vi "Dependencies.vi"   [LabVIEW 2009]
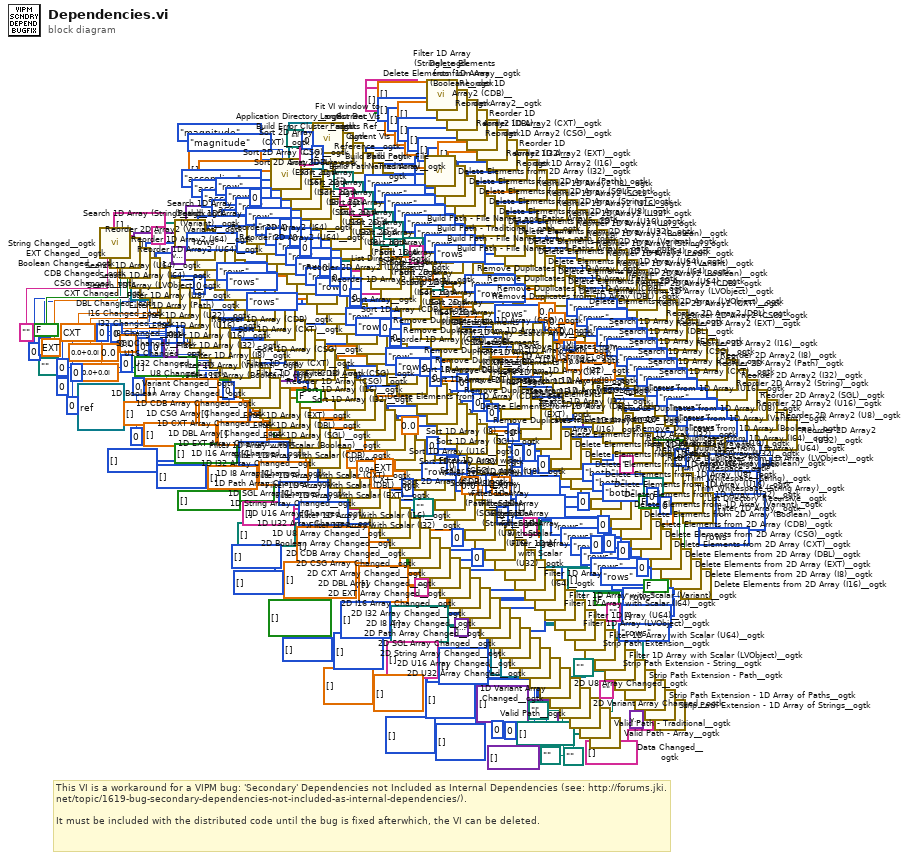
[diagram p0: block diagram]
diagram:
  # "This VI is a workaround for a VIPM bug: 'Secondary' Dependencies not Included as Internal Dependencies (see: http://forums.jki.net/topic/1619-bug-secondary-dependencies-not-included-as-internal-dependencies/).\n\nIt must be included with the distributed code until the bug is fixed afterwhich, the VI can be deleted."
  n1 = call <userlib>:"String Changed__ogtk.vi"("String"="") -> ()  [unwired: 1 out]
  n2 = call <userlib>:"EXT Changed__ogtk.vi"("EXT"=ext 0.0) -> ()  [unwired: 1 out]
  n3 = call <userlib>:"Boolean Changed__ogtk.vi"("Boolean"=FALSE) -> ()  [unwired: 1 out]
  n4 = call <userlib>:"CDB Changed__ogtk.vi"("CDB"=cdb 0.0+0.0i) -> ()  [unwired: 1 out]
  n5 = call <userlib>:"CSG Changed__ogtk.vi"("CSG"=csg 0.0+0.0i) -> ()  [unwired: 1 out]
  n6 = call <userlib>:"CXT Changed__ogtk.vi"("CXT"=cxt 0.0+0.0i) -> ()  [unwired: 1 out]
  n7 = call <userlib>:"DBL Changed__ogtk.vi"("DBL"=0.0) -> ()  [unwired: 1 out]
  n8 = call <userlib>:"I16 Changed__ogtk.vi"("I16"=i16 0) -> ()  [unwired: 1 out]
  n9 = call <userlib>:"Search 1D Array (String)__ogtk.vi"("Array"=string[] [], "Element Data"="", "Start Index (0)"=0) -> ()  [unwired: 6 in, 1 out]
  n10 = call <userlib>:"I32 Changed__ogtk.vi"("I32"=0) -> ()  [unwired: 1 out]
  n11 = call <userlib>:"Search 1D Array (Path)__ogtk.vi"("Array"=path[] [], "Element Data"=path "", "Start Index (0)"=0) -> ()  [unwired: 6 in, 1 out]
  n12 = call <userlib>:"I8 Changed__ogtk.vi"("I8"=i8 0) -> ()  [unwired: 1 out]
  n13 = call <userlib>:"Search 1D Array (Variant)__ogtk.vi"("Array"=variant[] [], "Element Data"=variant, "Start Index (0)"=0) -> ()  [unwired: 6 in, 1 out]
  n14 = call <userlib>:"SGL Changed__ogtk.vi"("SGL"=sgl 0.0) -> ()  [unwired: 1 out]
  n15 = call <userlib>:"Search 1D Array (U64)__ogtk.vi"("Array"=u64[] [], "Element Data"=u64 0, "Start Index (0)"=0) -> ()  [unwired: 6 in, 1 out]
  n16 = call <userlib>:"U16 Changed__ogtk.vi"("U16"=u16 0) -> ()  [unwired: 1 out]
  n17 = call <userlib>:"Search 1D Array (I64)__ogtk.vi"("Array"=i64[] [], "Element Data"=i64 0, "Start Index (0)"=0) -> ()  [unwired: 6 in, 1 out]
  n18 = call <userlib>:"U32 Changed__ogtk.vi"("U32"=u32 0) -> ()  [unwired: 1 out]
  n19 = call <userlib>:"Search 1D Array (LVObject)__ogtk.vi"("Array"=refnum<class>[] [], "Element Data"=refnum<class> refnum, "Start Index (0)"=0) -> ()  [unwired: 6 in, 1 out]
  n20 = call <userlib>:"U8 Changed__ogtk.vi"("U8"=u8 0) -> ()  [unwired: 1 out]
  n21 = call <userlib>:"Filter 1D Array (U8)__ogtk.vi"("items to filter"=u8[] [], "array"=u8[] []) -> ()  [unwired: 4 in, 2 out]
  n22 = call <userlib>:"Variant Changed__ogtk.vi"("Variant"=variant) -> ()  [unwired: 1 out]
  n23 = call <userlib>:"Filter 1D Array (Path)__ogtk.vi"("items to filter"=path[] [], "array"=path[] []) -> ()  [unwired: 4 in, 2 out]
  n24 = call <userlib>:"Reorder 2D Array2 (Variant)__ogtk.vi"("reorder (rows)"=enum16{"rows", "columns"}."rows", "indices"=i32[] [], "array"=variant[][] []) -> ()  [unwired: 8 in, 1 out]
  n25 = call <userlib>:"1D Boolean Array Changed__ogtk.vi"("1D Boolean Array"=bool[] []) -> ()  [unwired: 1 out]
  n26 = call <userlib>:"Filter 1D Array (U32)__ogtk.vi"("items to filter"=u32[] [], "array"=u32[] []) -> ()  [unwired: 4 in, 2 out]
  n27 = call <userlib>:"Reorder 1D Array2 (I64)__ogtk.vi"("indices"=i32[] [], "array"=i64[] []) -> ()  [unwired: 9 in, 1 out]
  n28 = call <userlib>:"1D CDB Array Changed__ogtk.vi"("1D CDB Array"=cdb[] []) -> ()  [unwired: 1 out]
  n29 = call <userlib>:"Filter 1D Array (U16)__ogtk.vi"("items to filter"=u16[] [], "array"=u16[] []) -> ()  [unwired: 4 in, 2 out]
  n30 = call <userlib>:"Reorder 1D Array2 (U64)__ogtk.vi"("indices"=i32[] [], "array"=u64[] []) -> ()  [unwired: 9 in, 1 out]
  n31 = call <userlib>:"1D CSG Array Changed__ogtk.vi"("1D CSG Array"=csg[] []) -> ()  [unwired: 1 out]
  n32 = call <userlib>:"Sort 2D Array (CXT)__ogtk.vi"("Column/Row to Sort By"=u32 0, "Method (magnitude)"=enum16{"real", "imaginary", "magnitude"}."magnitude", "Sort By in"=enum16{"row", "column"}."row", "Order"=enum16{"ascending", "descending"}."ascending", "Array in"=cxt[][] []) -> ()  [unwired: 3 in, 4 out]
  n33 = call <userlib>:"Filter 1D Array (I16)__ogtk.vi"("items to filter"=i16[] [], "array"=i16[] []) -> ()  [unwired: 4 in, 2 out]
  n34 = call <userlib>:"Reorder 2D Array2 (I64)__ogtk.vi"("reorder (rows)"=enum16{"rows", "columns"}."rows", "indices"=i32[] [], "array"=i64[][] []) -> ()  [unwired: 8 in, 1 out]
  n35 = call <userlib>:"1D CXT Array Changed__ogtk.vi"("1D CXT Array"=cxt[] []) -> ()  [unwired: 1 out]
  n36 = call <userlib>:"Sort 2D Array (CSG)__ogtk.vi"("Column/Row to Sort By"=u32 0, "Method (magnitude)"=enum16{"real", "imaginary", "magnitude"}."magnitude", "Sort By in"=enum16{"row", "column"}."row", "Order"=enum16{"ascending", "descending"}."ascending", "Array in"=csg[][] []) -> ()  [unwired: 3 in, 4 out]
  n37 = call <userlib>:"Filter 1D Array (I32)__ogtk.vi"("items to filter"=i32[] [], "array"=i32[] []) -> ()  [unwired: 4 in, 2 out]
  n38 = call <userlib>:"Reorder 2D Array2 (U64)__ogtk.vi"("reorder (rows)"=enum16{"rows", "columns"}."rows", "indices"=i32[] [], "array"=u64[][] []) -> ()  [unwired: 8 in, 1 out]
  n39 = call <userlib>:"1D DBL Array Changed__ogtk.vi"("1D DBL Array"=dbl[] []) -> ()  [unwired: 1 out]
  n40 = call <userlib>:"Sort 2D Array (DBL)__ogtk.vi"("Column/Row to Sort By"=u32 0, "Sort By in"=enum16{"row", "column"}."row", "Order"=enum16{"ascending", "descending"}."ascending", "Array in"=dbl[][] []) -> ()  [unwired: 4 in, 4 out]
  n41 = call <userlib>:"Filter 1D Array (I8)__ogtk.vi"("items to filter"=i8[] [], "array"=i8[] []) -> ()  [unwired: 4 in, 2 out]
  n42 = call <userlib>:"Reorder 1D Array2 (LVObject)__ogtk.vi"("indices"=i32[] [], "array"=refnum<class>[] []) -> ()  [unwired: 9 in, 1 out]
  n43 = call <userlib>:"1D EXT Array Changed__ogtk.vi"("1D EXT Array"=ext[] []) -> ()  [unwired: 1 out]
  n44 = call <userlib>:"Sort 2D Array (EXT)__ogtk.vi"("Column/Row to Sort By"=u32 0, "Sort By in"=enum16{"row", "column"}."row", "Order"=enum16{"ascending", "descending"}."ascending", "Array in"=ext[][] []) -> ()  [unwired: 4 in, 4 out]
  n45 = call <userlib>:"Filter 1D Array (Variant)__ogtk.vi"("items to filter"=variant[] [], "array"=variant[] []) -> ()  [unwired: 4 in, 2 out]
  n46 = call <userlib>:"Reorder 2D Array2 (LVObject)__ogtk.vi"("reorder (rows)"=enum16{"rows", "columns"}."rows", "indices"=i32[] [], "array"=refnum<class>[][] []) -> ()  [unwired: 8 in, 1 out]
  n47 = call <userlib>:"1D I16 Array Changed__ogtk.vi"("1D I16 Array"=i16[] []) -> ()  [unwired: 1 out]
  n48 = call <userlib>:"Sort 2D Array (I16)__ogtk.vi"("Column/Row to Sort By"=u32 0, "Sort By in"=enum16{"row", "column"}."row", "Order"=enum16{"ascending", "descending"}."ascending", "Array in"=i16[][] []) -> ()  [unwired: 4 in, 4 out]
  n49 = call <userlib>:"Application Directory__ogtk.vi"("Relative path (.)"=path "") -> ()  [unwired: 1 out]
  n50 = call <userlib>:"Filter 1D Array (Boolean)__ogtk.vi"("items to filter"=bool[] [], "array"=bool[] []) -> ()  [unwired: 4 in, 2 out]
  n51 = call-poly <userlib>:"Sort Array__ogtk.vi"("Order"=enum16{"ascending", "descending"}."ascending", "Array in"=dbl[] []) -> ()  [unwired: 8 in, 2 out]
  n52 = call <userlib>:"1D I32 Array Changed__ogtk.vi"("1D I32 Array"=i32[] []) -> ()  [unwired: 1 out]
  n53 = call <userlib>:"Sort 2D Array (I32)__ogtk.vi"("Column/Row to Sort By"=u32 0, "Sort By in"=enum16{"row", "column"}."row", "Order"=enum16{"ascending", "descending"}."ascending", "Array in"=i32[][] []) -> ()  [unwired: 4 in, 4 out]
  n54 = call <userlib>:"Build Error Cluster__ogtk.vi"("String to Prepend to source (\"\")"="" ("String to Prepend to source (\"\")"), "code"=0) -> ()  [unwired: 1 out]
  n55 = call <userlib>:"Filter 1D Array (CXT)__ogtk.vi"("items to filter"=cxt[] [], "array"=cxt[] []) -> ()  [unwired: 4 in, 2 out]
  n56 = call <userlib>:"Sort 1D Array (CDB)__ogtk.vi"("Method (magnitude)"=enum16{"real", "imaginary", "magnitude"}."magnitude", "Order"=enum16{"ascending", "descending"}."ascending", "Array in"=cdb[] []) -> ()  [unwired: 7 in, 2 out]
  n57 = call <userlib>:"1D I8 Array Changed__ogtk.vi"("1D I8 Array"=i8[] []) -> ()  [unwired: 1 out]
  n58 = call <userlib>:"Sort 2D Array (I8)__ogtk.vi"("Column/Row to Sort By"=u32 0, "Sort By in"=enum16{"row", "column"}."row", "Order"=enum16{"ascending", "descending"}."ascending", "Array in"=i8[][] []) -> ()  [unwired: 4 in, 4 out]
  n59 = call <userlib>:"Fit VI window to Largest Dec__ogtk.vi"("error in (no error)"=errorcluster {"status"=FALSE, "code"=0, "source"=""}, "border spacing (2 px)"=2, "VI Ref (calling VI)"=refnum<vi> refnum) -> ()  [unwired: 3 in, 2 out]
  n60 = call <userlib>:"Filter 1D Array (CDB)__ogtk.vi"("items to filter"=cdb[] [], "array"=cdb[] []) -> ()  [unwired: 4 in, 2 out]
  n61 = call <userlib>:"Reorder 1D Array (CDB)__ogtk.vi"("Sorted Pointers in"=i32[] [], "Array in"=cdb[] []) -> ()  [unwired: 8 in, 2 out]
  n62 = call <userlib>:"1D Path Array Changed__ogtk.vi"("1D Path Array"=path[] []) -> ()  [unwired: 1 out]
  n63 = call <userlib>:"Sort 2D Array (SGL)__ogtk.vi"("Column/Row to Sort By"=u32 0, "Sort By in"=enum16{"row", "column"}."row", "Order"=enum16{"ascending", "descending"}."ascending", "Array in"=sgl[][] []) -> ()  [unwired: 4 in, 4 out]
  n64 = call <userlib>:"Current VIs Parents Ref__ogtk.vi"() -> ()  [unwired: 2 in, 1 out]
  n65 = call <userlib>:"Filter 1D Array (CSG)__ogtk.vi"("items to filter"=csg[] [], "array"=csg[] []) -> ()  [unwired: 4 in, 2 out]
  n66 = call <userlib>:"Sort 1D Array (CXT)__ogtk.vi"("Method (magnitude)"=enum16{"real", "imaginary", "magnitude"}."magnitude", "Order"=enum16{"ascending", "descending"}."ascending", "Array in"=cxt[] []) -> ()  [unwired: 7 in, 2 out]
  n67 = call <userlib>:"1D SGL Array Changed__ogtk.vi"("1D SGL Array"=sgl[] []) -> ()  [unwired: 1 out]
  n68 = call <userlib>:"Sort 2D Array (U16)__ogtk.vi"("Column/Row to Sort By"=u32 0, "Sort By in"=enum16{"row", "column"}."row", "Order"=enum16{"ascending", "descending"}."ascending", "Array in"=u16[][] []) -> ()  [unwired: 4 in, 4 out]
  n69 = call <userlib>:"Current VIs Reference__ogtk.vi"() -> ()  [unwired: 5 in, 1 out]
  n70 = call <userlib>:"Filter 1D Array (EXT)__ogtk.vi"("items to filter"=ext[] [], "array"=ext[] []) -> ()  [unwired: 4 in, 2 out]
  n71 = call <userlib>:"Reorder 1D Array (CXT)__ogtk.vi"("Sorted Pointers in"=i32[] [], "Array in"=cxt[] []) -> ()  [unwired: 8 in, 2 out]
  n72 = call <userlib>:"1D String Array Changed__ogtk.vi"("1D String Array"=string[] []) -> ()  [unwired: 1 out]
  n73 = call <userlib>:"Sort 2D Array (U32)__ogtk.vi"("Column/Row to Sort By"=u32 0, "Sort By in"=enum16{"row", "column"}."row", "Order"=enum16{"ascending", "descending"}."ascending", "Array in"=u32[][] []) -> ()  [unwired: 4 in, 4 out]
  n74 = call-poly <userlib>:"Build Path__ogtk.vi"("name or relative path"="", "base path"=path "") -> ()  [unwired: 1 out]
  n75 = call <userlib>:"Filter 1D Array (DBL)__ogtk.vi"("items to filter"=dbl[] [], "array"=dbl[] []) -> ()  [unwired: 4 in, 2 out]
  n76 = call <userlib>:"Sort 1D Array (CSG)__ogtk.vi"("Method (magnitude)"=enum16{"real", "imaginary", "magnitude"}."magnitude", "Order"=enum16{"ascending", "descending"}."ascending", "Array in"=csg[] []) -> ()  [unwired: 7 in, 2 out]
  n77 = call <userlib>:"1D U16 Array Changed__ogtk.vi"("1D U16 Array"=u16[] []) -> ()  [unwired: 1 out]
  n78 = call <userlib>:"Sort 2D Array (U8)__ogtk.vi"("Column/Row to Sort By"=u32 0, "Sort By in"=enum16{"row", "column"}."row", "Order"=enum16{"ascending", "descending"}."ascending", "Array in"=u8[][] []) -> ()  [unwired: 4 in, 4 out]
  n79 = call <userlib>:"Build Path - Traditional__ogtk.vi"("name or relative path"="", "base path"=path "") -> ()  [unwired: 1 out]
  n80 = call <userlib>:"Filter 1D Array (SGL)__ogtk.vi"("items to filter"=sgl[] [], "array"=sgl[] []) -> ()  [unwired: 4 in, 2 out]
  n81 = call <userlib>:"Reorder 1D Array (CSG)__ogtk.vi"("Sorted Pointers in"=i32[] [], "Array in"=csg[] []) -> ()  [unwired: 8 in, 2 out]
  n82 = call <userlib>:"1D U32 Array Changed__ogtk.vi"("1D U32 Array"=u32[] []) -> ()  [unwired: 1 out]
  n83 = call <userlib>:"Sort 1D Array (Path)__ogtk.vi"("Order"=enum16{"ascending", "descending"}."ascending", "Array in"=path[] []) -> ()  [unwired: 8 in, 2 out]
  n84 = call <userlib>:"Build Path - File Names Array__ogtk.vi"("name or relative path"=string[] [], "base path"=path "") -> ()  [unwired: 1 out]
  n85 = call <userlib>:"Filter 1D Array with Scalar (Boolean)__ogtk.vi"("items to filter"=FALSE, "array"=bool[] []) -> ()  [unwired: 4 in, 2 out]
  n86 = call <userlib>:"Sort 1D Array (DBL)__ogtk.vi"("Order"=enum16{"ascending", "descending"}."ascending", "Array in"=dbl[] []) -> ()  [unwired: 8 in, 2 out]
  n87 = call <userlib>:"1D U8 Array Changed__ogtk.vi"("1D U8 Array"=u8[] []) -> ()  [unwired: 1 out]
  n88 = call <userlib>:"Sort 1D Array (String)__ogtk.vi"("Order"=enum16{"ascending", "descending"}."ascending", "Array in"=string[] []) -> ()  [unwired: 8 in, 2 out]
  n89 = call <userlib>:"Build Path - File Names and Paths Arrays__ogtk.vi"("name or relative path"=string[] [], "base path"=path[] []) -> ()  [unwired: 1 out]
  n90 = call <userlib>:"Filter 1D Array with Scalar (CDB)__ogtk.vi"("items to filter"=cdb 0.0+0.0i, "array"=cdb[] []) -> ()  [unwired: 4 in, 2 out]
  n91 = call <userlib>:"Sort 1D Array (EXT)__ogtk.vi"("Order"=enum16{"ascending", "descending"}."ascending", "Array in"=ext[] []) -> ()  [unwired: 8 in, 2 out]
  n92 = call <userlib>:"2D Boolean Array Changed__ogtk.vi"("2D Boolean Array"=bool[][] []) -> ()  [unwired: 1 out]
  n93 = call <userlib>:"Sort 2D Array (Path)__ogtk.vi"("Column/Row to Sort By"=u32 0, "Sort By in"=enum16{"row", "column"}."row", "Order"=enum16{"ascending", "descending"}."ascending", "Array in"=path[][] []) -> ()  [unwired: 4 in, 4 out]
  n94 = call <userlib>:"Build Path - Traditional - path__ogtk.vi"("name or relative path"=path "", "base path"=path "") -> ()  [unwired: 1 out]
  n95 = call <userlib>:"Filter 1D Array with Scalar (CSG)__ogtk.vi"("items to filter"=csg 0.0+0.0i, "array"=csg[] []) -> ()  [unwired: 4 in, 2 out]
  n96 = call <userlib>:"Sort 1D Array (I16)__ogtk.vi"("Order"=enum16{"ascending", "descending"}."ascending", "Array in"=i16[] []) -> ()  [unwired: 8 in, 2 out]
  n97 = call <userlib>:"2D CDB Array Changed__ogtk.vi"("2D CDB Array"=cdb[][] []) -> ()  [unwired: 1 out]
  n98 = call <userlib>:"Sort 2D Array (String)__ogtk.vi"("Column/Row to Sort By"=u32 0, "Sort By in"=enum16{"row", "column"}."row", "Order"=enum16{"ascending", "descending"}."ascending", "Array in"=string[][] []) -> ()  [unwired: 4 in, 4 out]
  n99 = call <userlib>:"Build Path - File Names Array - path__ogtk.vi"("name or relative path"=path[] [], "base path"=path "") -> ()  [unwired: 1 out]
  n100 = call <userlib>:"Filter 1D Array with Scalar (CXT)__ogtk.vi"("items to filter"=cxt 0.0+0.0i, "array"=cxt[] []) -> ()  [unwired: 4 in, 2 out]
  n101 = call <userlib>:"Sort 1D Array (I32)__ogtk.vi"("Order"=enum16{"ascending", "descending"}."ascending", "Array in"=i32[] []) -> ()  [unwired: 8 in, 2 out]
  n102 = call <userlib>:"2D CSG Array Changed__ogtk.vi"("2D CSG Array"=csg[][] []) -> ()  [unwired: 1 out]
  n103 = call <userlib>:"Sort 1D Array (I64)__ogtk.vi"("Order"=enum16{"ascending", "descending"}."ascending", "Array in"=i64[] []) -> ()  [unwired: 8 in, 2 out]
  n104 = call <userlib>:"Build Path - File Names and Paths Arrays - path__ogtk.vi"("name or relative path"=path[] [], "base path"=path[] []) -> ()  [unwired: 1 out]
  n105 = call <userlib>:"Delete Elements from 2D Array (I32)__ogtk.vi"("delete (rows or columns)"=enum16{"rows", "columns"}."rows", "indices"=i32[] [], "array"=i32[][] []) -> ()  [unwired: 7 in, 2 out]
  n106 = call <userlib>:"Filter 1D Array with Scalar (DBL)__ogtk.vi"("items to filter"=0.0, "array"=dbl[] []) -> ()  [unwired: 4 in, 2 out]
  n107 = call <userlib>:"Filter 1D Array (String)__ogtk.vi"("items to filter"=string[] [], "array"=string[] []) -> ()  [unwired: 4 in, 2 out]
  n108 = call <userlib>:"Sort 1D Array (I8)__ogtk.vi"("Order"=enum16{"ascending", "descending"}."ascending", "Array in"=i8[] []) -> ()  [unwired: 8 in, 2 out]
  n109 = call <userlib>:"2D CXT Array Changed__ogtk.vi"("2D CXT Array"=cxt[][] []) -> ()  [unwired: 1 out]
  n110 = call <userlib>:"Sort 1D Array (U64)__ogtk.vi"("Order"=enum16{"ascending", "descending"}."ascending", "Array in"=u64[] []) -> ()  [unwired: 8 in, 2 out]
  n111 = call <userlib>:"List Directory__ogtk.vi"("error in (no error)"=errorcluster {"status"=FALSE, "code"=0, "source"=""}, "pattern"="", "directory path"=path "") -> ()  [unwired: 1 in, 4 out]
  n112 = call <userlib>:"Delete Elements from 2D Array (Path)__ogtk.vi"("delete (rows or columns)"=enum16{"rows", "columns"}."rows", "indices"=i32[] [], "array"=path[][] []) -> ()  [unwired: 7 in, 2 out]
  n113 = call <userlib>:"Filter 1D Array with Scalar (EXT)__ogtk.vi"("items to filter"=ext 0.0, "array"=ext[] []) -> ()  [unwired: 4 in, 2 out]
  n114 = call-poly <userlib>:"Delete Elements from Array__ogtk.vi"("indices"=i32[] [], "array"=dbl[] []) -> ()  [unwired: 8 in, 2 out]
  n115 = call <userlib>:"Sort 1D Array (SGL)__ogtk.vi"("Order"=enum16{"ascending", "descending"}."ascending", "Array in"=sgl[] []) -> ()  [unwired: 8 in, 2 out]
  n116 = call <userlib>:"2D DBL Array Changed__ogtk.vi"("2D DBL Array"=dbl[][] []) -> ()  [unwired: 1 out]
  n117 = call <userlib>:"Sort 2D Array (I64)__ogtk.vi"("Column/Row to Sort By"=u32 0, "Sort By in"=enum16{"row", "column"}."row", "Order"=enum16{"ascending", "descending"}."ascending", "Array in"=i64[][] []) -> ()  [unwired: 4 in, 4 out]
  n118 = call-poly <userlib>:"Remove Duplicates from 1D Array__ogtk.vi"("Input Array"=dbl[] []) -> ()  [unwired: 2 out]
  n119 = call <userlib>:"Delete Elements from 2D Array (SGL)__ogtk.vi"("delete (rows or columns)"=enum16{"rows", "columns"}."rows", "indices"=i32[] [], "array"=sgl[][] []) -> ()  [unwired: 7 in, 2 out]
  n120 = call <userlib>:"Filter 1D Array with Scalar (I8)__ogtk.vi"("items to filter"=i8 0, "array"=i8[] []) -> ()  [unwired: 4 in, 2 out]
  n121 = call <userlib>:"Delete Elements from 1D Array (Boolean)__ogtk.vi"("indices"=i32[] [], "array"=bool[] []) -> ()  [unwired: 8 in, 2 out]
  n122 = call <userlib>:"Sort 1D Array (U16)__ogtk.vi"("Order"=enum16{"ascending", "descending"}."ascending", "Array in"=u16[] []) -> ()  [unwired: 8 in, 2 out]
  n123 = call <userlib>:"2D EXT Array Changed__ogtk.vi"("2D EXT Array"=ext[][] []) -> ()  [unwired: 1 out]
  n124 = call <userlib>:"Sort 2D Array (U64)__ogtk.vi"("Column/Row to Sort By"=u32 0, "Sort By in"=enum16{"row", "column"}."row", "Order"=enum16{"ascending", "descending"}."ascending", "Array in"=u64[][] []) -> ()  [unwired: 4 in, 4 out]
  n125 = call <userlib>:"Remove Duplicates from 1D Array (Path)__ogtk.vi"("Input Array"=path[] []) -> ()  [unwired: 2 out]
  n126 = call <userlib>:"Delete Elements from 2D Array (String)__ogtk.vi"("delete (rows or columns)"=enum16{"rows", "columns"}."rows", "indices"=i32[] [], "array"=string[][] []) -> ()  [unwired: 7 in, 2 out]
  n127 = call <userlib>:"Filter 1D Array with Scalar (I16)__ogtk.vi"("items to filter"=i16 0, "array"=i16[] []) -> ()  [unwired: 4 in, 2 out]
  n128 = call-poly <userlib>:"Reorder Array2__ogtk.vi"("indices"=i32[] [], "array"=dbl[] []) -> ()  [unwired: 9 in, 1 out]
  n129 = call <userlib>:"Sort 1D Array (U32)__ogtk.vi"("Order"=enum16{"ascending", "descending"}."ascending", "Array in"=u32[] []) -> ()  [unwired: 8 in, 2 out]
  n130 = call <userlib>:"2D I16 Array Changed__ogtk.vi"("2D I16 Array"=i16[][] []) -> ()  [unwired: 1 out]
  n131 = call <userlib>:"Delete Elements from 1D Array (CDB)__ogtk.vi"("indices"=i32[] [], "array"=cdb[] []) -> ()  [unwired: 8 in, 2 out]
  n132 = call <userlib>:"Remove Duplicates from 1D Array (CDB)__ogtk.vi"("Input Array"=cdb[] []) -> ()  [unwired: 2 out]
  n133 = call <userlib>:"Delete Elements from 2D Array (U8)__ogtk.vi"("delete (rows or columns)"=enum16{"rows", "columns"}."rows", "indices"=i32[] [], "array"=u8[][] []) -> ()  [unwired: 7 in, 2 out]
  n134 = call <userlib>:"Filter 1D Array with Scalar (I32)__ogtk.vi"("items to filter"=0, "array"=i32[] []) -> ()  [unwired: 4 in, 2 out]
  n135 = call <userlib>:"Reorder 1D Array2 (CDB)__ogtk.vi"("indices"=i32[] [], "array"=cdb[] []) -> ()  [unwired: 9 in, 1 out]
  n136 = call <userlib>:"Sort 1D Array (U8)__ogtk.vi"("Order"=enum16{"ascending", "descending"}."ascending", "Array in"=u8[] []) -> ()  [unwired: 8 in, 2 out]
  n137 = call <userlib>:"2D I32 Array Changed__ogtk.vi"("2D I32 Array"=i32[][] []) -> ()  [unwired: 1 out]
  n138 = call <userlib>:"Delete Elements from 1D Array (CSG)__ogtk.vi"("indices"=i32[] [], "array"=csg[] []) -> ()  [unwired: 8 in, 2 out]
  n139 = call <userlib>:"Remove Duplicates from 1D Array (CSG)__ogtk.vi"("Input Array"=csg[] []) -> ()  [unwired: 2 out]
  n140 = call <userlib>:"Delete Elements from 2D Array (U16)__ogtk.vi"("delete (rows or columns)"=enum16{"rows", "columns"}."rows", "indices"=i32[] [], "array"=u16[][] []) -> ()  [unwired: 7 in, 2 out]
  n141 = call <userlib>:"Filter 1D Array with Scalar (Path)__ogtk.vi"("items to filter"=path "", "array"=path[] []) -> ()  [unwired: 4 in, 2 out]
  n142 = call <userlib>:"Reorder 1D Array2 (CXT)__ogtk.vi"("indices"=i32[] [], "array"=cxt[] []) -> ()  [unwired: 9 in, 1 out]
  n143 = call <userlib>:"Sort 2D Array (CDB)__ogtk.vi"("Column/Row to Sort By"=u32 0, "Method (magnitude)"=enum16{"real", "imaginary", "magnitude"}."magnitude", "Sort By in"=enum16{"row", "column"}."row", "Order"=enum16{"ascending", "descending"}."ascending", "Array in"=cdb[][] []) -> ()  [unwired: 3 in, 4 out]
  n144 = call <userlib>:"2D I8 Array Changed__ogtk.vi"("2D I8 Array"=i8[][] []) -> ()  [unwired: 1 out]
  n145 = call <userlib>:"Delete Elements from 1D Array (DBL)__ogtk.vi"("indices"=i32[] [], "array"=dbl[] []) -> ()  [unwired: 8 in, 2 out]
  n146 = call <userlib>:"Remove Duplicates from 1D Array (CXT)__ogtk.vi"("Input Array"=cxt[] []) -> ()  [unwired: 2 out]
  n147 = call <userlib>:"Delete Elements from 2D Array (U32)__ogtk.vi"("delete (rows or columns)"=enum16{"rows", "columns"}."rows", "indices"=i32[] [], "array"=u32[][] []) -> ()  [unwired: 7 in, 2 out]
  n148 = call <userlib>:"Filter 1D Array with Scalar (SGL)__ogtk.vi"("items to filter"=sgl 0.0, "array"=sgl[] []) -> ()  [unwired: 4 in, 2 out]
  n149 = call <userlib>:"Reorder 1D Array2 (CSG)__ogtk.vi"("indices"=i32[] [], "array"=csg[] []) -> ()  [unwired: 9 in, 1 out]
  n150 = call <userlib>:"2D Path Array Changed__ogtk.vi"("2D Path Array"=path[][] []) -> ()  [unwired: 1 out]
  n151 = call <userlib>:"Delete Elements from 1D Array (CXT)__ogtk.vi"("indices"=i32[] [], "array"=cxt[] []) -> ()  [unwired: 8 in, 2 out]
  n152 = call <userlib>:"Remove Duplicates from 1D Array (DBL)__ogtk.vi"("Input Array"=dbl[] []) -> ()  [unwired: 2 out]
  n153 = call <userlib>:"Delete Elements from 2D Array (Variant)__ogtk.vi"("delete (rows or columns)"=enum16{"rows", "columns"}."rows", "indices"=i32[] [], "array"=variant[][] []) -> ()  [unwired: 7 in, 2 out]
  n154 = call <userlib>:"Filter 1D Array with Scalar (String)__ogtk.vi"("items to filter"="", "array"=string[] []) -> ()  [unwired: 4 in, 2 out]
  n155 = call <userlib>:"Reorder 1D Array2 (DBL)__ogtk.vi"("indices"=i32[] [], "array"=dbl[] []) -> ()  [unwired: 9 in, 1 out]
  n156 = call <userlib>:"2D SGL Array Changed__ogtk.vi"("2D SGL Array"=sgl[][] []) -> ()  [unwired: 1 out]
  n157 = call <userlib>:"Delete Elements from 1D Array (EXT)__ogtk.vi"("indices"=i32[] [], "array"=ext[] []) -> ()  [unwired: 8 in, 2 out]
  n158 = call <userlib>:"Remove Duplicates from 1D Array (EXT)__ogtk.vi"("Input Array"=ext[] []) -> ()  [unwired: 2 out]
  n159 = call <userlib>:"Delete Elements from 1D Array (I64)__ogtk.vi"("indices"=i32[] [], "array"=i64[] []) -> ()  [unwired: 8 in, 2 out]
  n160 = call <userlib>:"Filter 1D Array with Scalar (U8)__ogtk.vi"("items to filter"=u8 0, "array"=u8[] []) -> ()  [unwired: 4 in, 2 out]
  n161 = call <userlib>:"Reorder 1D Array2 (EXT)__ogtk.vi"("indices"=i32[] [], "array"=ext[] []) -> ()  [unwired: 9 in, 1 out]
  n162 = call <userlib>:"2D String Array Changed__ogtk.vi"("2D String Array"=string[][] []) -> ()  [unwired: 1 out]
  n163 = call <userlib>:"Delete Elements from 1D Array (I8)__ogtk.vi"("indices"=i32[] [], "array"=i8[] []) -> ()  [unwired: 8 in, 2 out]
  n164 = call <userlib>:"Remove Duplicates from 1D Array (I16)__ogtk.vi"("Input Array"=i16[] []) -> ()  [unwired: 2 out]
  n165 = call <userlib>:"Delete Elements from 1D Array (U64)__ogtk.vi"("indices"=i32[] [], "array"=u64[] []) -> ()  [unwired: 8 in, 2 out]
  n166 = call <userlib>:"Filter 1D Array with Scalar (U16)__ogtk.vi"("items to filter"=u16 0, "array"=u16[] []) -> ()  [unwired: 4 in, 2 out]
  n167 = call <userlib>:"Reorder 1D Array2 (I16)__ogtk.vi"("indices"=i32[] [], "array"=i16[] []) -> ()  [unwired: 9 in, 1 out]
  n168 = call <userlib>:"2D U16 Array Changed__ogtk.vi"("2D U16 Array"=u16[][] []) -> ()  [unwired: 1 out]
  n169 = call <userlib>:"Delete Elements from 1D Array (I16)__ogtk.vi"("indices"=i32[] [], "array"=i16[] []) -> ()  [unwired: 8 in, 2 out]
  n170 = call <userlib>:"Remove Duplicates from 1D Array (I32)__ogtk.vi"("Input Array"=i32[] []) -> ()  [unwired: 2 out]
  n171 = call <userlib>:"Delete Elements from 2D Array (I64)__ogtk.vi"("delete (rows or columns)"=enum16{"rows", "columns"}."rows", "indices"=i32[] [], "array"=i64[][] []) -> ()  [unwired: 7 in, 2 out]
  n172 = call <userlib>:"Filter 1D Array with Scalar (U32)__ogtk.vi"("items to filter"=u32 0, "array"=u32[] []) -> ()  [unwired: 4 in, 2 out]
  n173 = call <userlib>:"Reorder 1D Array2 (I32)__ogtk.vi"("indices"=i32[] [], "array"=i32[] []) -> ()  [unwired: 9 in, 1 out]
  n174 = call <userlib>:"2D U32 Array Changed__ogtk.vi"("2D U32 Array"=u32[][] []) -> ()  [unwired: 1 out]
  n175 = call <userlib>:"Delete Elements from 1D Array (I32)__ogtk.vi"("indices"=i32[] [], "array"=i32[] []) -> ()  [unwired: 8 in, 2 out]
  n176 = call <userlib>:"Remove Duplicates from 1D Array (I8)__ogtk.vi"("Input Array"=i8[] []) -> ()  [unwired: 2 out]
  n177 = call <userlib>:"Delete Elements from 2D Array (U64)__ogtk.vi"("delete (rows or columns)"=enum16{"rows", "columns"}."rows", "indices"=i32[] [], "array"=u64[][] []) -> ()  [unwired: 7 in, 2 out]
  n178 = call <userlib>:"Filter 1D Array with Scalar (Variant)__ogtk.vi"("items to filter"=variant, "array"=variant[] []) -> ()  [unwired: 4 in, 2 out]
  n179 = call <userlib>:"Reorder 1D Array2 (I8)__ogtk.vi"("indices"=i32[] [], "array"=i8[] []) -> ()  [unwired: 9 in, 1 out]
  n180 = call <userlib>:"2D U8 Array Changed__ogtk.vi"("2D U8 Array"=u8[][] []) -> ()  [unwired: 1 out]
  n181 = call <userlib>:"Delete Elements from 1D Array (Path)__ogtk.vi"("indices"=i32[] [], "array"=path[] []) -> ()  [unwired: 8 in, 2 out]
  n182 = call <userlib>:"Remove Duplicates from 1D Array (SGL)__ogtk.vi"("Input Array"=sgl[] []) -> ()  [unwired: 2 out]
  n183 = call <userlib>:"Delete Elements from 1D Array (LVObject)__ogtk.vi"("indices"=i32[] [], "array"=refnum<class>[] []) -> ()  [unwired: 8 in, 2 out]
  n184 = call <userlib>:"Filter 1D Array (I64)__ogtk.vi"("items to filter"=i64[] [], "array"=i64[] []) -> ()  [unwired: 4 in, 2 out]
  n185 = call <userlib>:"Reorder 1D Array2 (SGL)__ogtk.vi"("indices"=i32[] [], "array"=sgl[] []) -> ()  [unwired: 9 in, 1 out]
  n186 = call <userlib>:"1D Variant Array Changed__ogtk.vi"("1D Variant Array"=variant[] []) -> ()  [unwired: 1 out]
  n187 = call <userlib>:"Delete Elements from 1D Array (SGL)__ogtk.vi"("indices"=i32[] [], "array"=sgl[] []) -> ()  [unwired: 8 in, 2 out]
  n188 = call <userlib>:"Remove Duplicates from 1D Array (String)__ogtk.vi"("Input Array"=string[] []) -> ()  [unwired: 2 out]
  n189 = call <userlib>:"Delete Elements from 2D Array (LVObject)__ogtk.vi"("delete (rows or columns)"=enum16{"rows", "columns"}."rows", "indices"=i32[] [], "array"=refnum<class>[][] []) -> ()  [unwired: 7 in, 2 out]
  n190 = call <userlib>:"Filter 1D Array (U64)__ogtk.vi"("items to filter"=u64[] [], "array"=u64[] []) -> ()  [unwired: 4 in, 2 out]
  n191 = call <userlib>:"Reorder 1D Array2 (U16)__ogtk.vi"("indices"=i32[] [], "array"=u16[] []) -> ()  [unwired: 9 in, 1 out]
  n192 = call <userlib>:"2D Variant Array Changed__ogtk.vi"("2D Variant Array"=variant[][] []) -> ()  [unwired: 1 out]
  n193 = call <userlib>:"Delete Elements from 1D Array (String)__ogtk.vi"("indices"=i32[] [], "array"=string[] []) -> ()  [unwired: 8 in, 2 out]
  n194 = call <userlib>:"Remove Duplicates from 1D Array (U16)__ogtk.vi"("Input Array"=u16[] []) -> ()  [unwired: 2 out]
  n195 = call-poly <userlib>:"Search Array__ogtk.vi"("Array"=dbl[] [], "Element Data"=0.0, "Start Index (0)"=0) -> ()  [unwired: 6 in, 1 out]
  n196 = call <userlib>:"Filter 1D Array with Scalar (I64)__ogtk.vi"("items to filter"=i64 0, "array"=i64[] []) -> ()  [unwired: 4 in, 2 out]
  n197 = call <userlib>:"Reorder 1D Array2 (U32)__ogtk.vi"("indices"=i32[] [], "array"=u32[] []) -> ()  [unwired: 9 in, 1 out]
  n198 = call-poly <userlib>:"Valid Path__ogtk.vi"("path"=path "") -> ()  [unwired: 1 out]
  n199 = call <userlib>:"Delete Elements from 1D Array (U8)__ogtk.vi"("indices"=i32[] [], "array"=u8[] []) -> ()  [unwired: 8 in, 2 out]
  n200 = call <userlib>:"Remove Duplicates from 1D Array (U32)__ogtk.vi"("Input Array"=u32[] []) -> ()  [unwired: 2 out]
  n201 = call <userlib>:"Search 1D Array (SGL)__ogtk.vi"("Array"=sgl[] [], "Element Data"=sgl 0.0, "Start Index (0)"=0) -> ()  [unwired: 6 in, 1 out]
  n202 = call <userlib>:"Filter 1D Array with Scalar (U64)__ogtk.vi"("items to filter"=u64 0, "array"=u64[] []) -> ()  [unwired: 4 in, 2 out]
  n203 = call <userlib>:"Reorder 1D Array2 (U8)__ogtk.vi"("indices"=i32[] [], "array"=u8[] []) -> ()  [unwired: 9 in, 1 out]
  n204 = call <userlib>:"Valid Path - Traditional__ogtk.vi"("path"=path "") -> ()  [unwired: 1 out]
  n205 = call <userlib>:"Delete Elements from 1D Array (U16)__ogtk.vi"("indices"=i32[] [], "array"=u16[] []) -> ()  [unwired: 8 in, 2 out]
  n206 = call <userlib>:"Remove Duplicates from 1D Array (U8)__ogtk.vi"("Input Array"=u8[] []) -> ()  [unwired: 2 out]
  n207 = call <userlib>:"Search 1D Array (DBL)__ogtk.vi"("Array"=dbl[] [], "Element Data"=0.0, "Start Index (0)"=0) -> ()  [unwired: 6 in, 1 out]
  n208 = call <userlib>:"Filter 1D Array (LVObject)__ogtk.vi"("items to filter"=refnum<class>[] [], "array"=refnum<class>[] []) -> ()  [unwired: 4 in, 2 out]
  n209 = call <userlib>:"Reorder 1D Array2 (Boolean)__ogtk.vi"("indices"=i32[] [], "array"=bool[] []) -> ()  [unwired: 9 in, 1 out]
  n210 = call <userlib>:"Valid Path - Array__ogtk.vi"("array of paths"=path[] []) -> ()  [unwired: 1 out]
  n211 = call <userlib>:"Delete Elements from 1D Array (U32)__ogtk.vi"("indices"=i32[] [], "array"=u32[] []) -> ()  [unwired: 8 in, 2 out]
  n212 = call <userlib>:"Remove Duplicates from 1D Array (Variant)__ogtk.vi"("Input Array"=variant[] []) -> ()  [unwired: 2 out]
  n213 = call <userlib>:"Search 1D Array (EXT)__ogtk.vi"("Array"=ext[] [], "Element Data"=ext 0.0, "Start Index (0)"=0) -> ()  [unwired: 6 in, 1 out]
  n214 = call <userlib>:"Filter 1D Array with Scalar (LVObject)__ogtk.vi"("items to filter"=refnum<class> refnum, "array"=refnum<class>[] []) -> ()  [unwired: 4 in, 2 out]
  n215 = call <userlib>:"Reorder 1D Array2 (String)__ogtk.vi"("indices"=i32[] [], "array"=string[] []) -> ()  [unwired: 9 in, 1 out]
  n216 = call <userlib>:"Delete Elements from 1D Array (Variant)__ogtk.vi"("indices"=i32[] [], "array"=variant[] []) -> ()  [unwired: 8 in, 2 out]
  n217 = call <userlib>:"Remove Duplicates from 1D Array (Boolean)__ogtk.vi"("Input Array"=bool[] []) -> ()  [unwired: 2 out]
  n218 = call <userlib>:"Search 1D Array (CSG)__ogtk.vi"("Array"=csg[] [], "Element Data"=csg 0.0+0.0i, "Start Index (0)"=0) -> ()  [unwired: 6 in, 1 out]
  n219 = call-poly <userlib>:"Strip Path Extension__ogtk.vi"("path"=path "") -> ()  [unwired: 2 out]
  n220 = call <userlib>:"Reorder 1D Array2 (Path)__ogtk.vi"("indices"=i32[] [], "array"=path[] []) -> ()  [unwired: 9 in, 1 out]
  n221 = call <userlib>:"Delete Elements from 2D Array (Boolean)__ogtk.vi"("delete (rows or columns)"=enum16{"rows", "columns"}."rows", "indices"=i32[] [], "array"=bool[][] []) -> ()  [unwired: 7 in, 2 out]
  n222 = call <userlib>:"Remove Duplicates from 1D Array (I64)__ogtk.vi"("Input Array"=i64[] []) -> ()  [unwired: 2 out]
  n223 = call <userlib>:"Search 1D Array (CDB)__ogtk.vi"("Array"=cdb[] [], "Element Data"=cdb 0.0+0.0i, "Start Index (0)"=0) -> ()  [unwired: 6 in, 1 out]
  n224 = call <userlib>:"Strip Path Extension - Path__ogtk.vi"("path"=path "") -> ()  [unwired: 2 out]
  n225 = call <userlib>:"Reorder 1D Array2 (Variant)__ogtk.vi"("indices"=i32[] [], "array"=variant[] []) -> ()  [unwired: 9 in, 1 out]
  n226 = call <userlib>:"Delete Elements from 2D Array (CDB)__ogtk.vi"("delete (rows or columns)"=enum16{"rows", "columns"}."rows", "indices"=i32[] [], "array"=cdb[][] []) -> ()  [unwired: 7 in, 2 out]
  n227 = call <userlib>:"Remove Duplicates from 1D Array (U64)__ogtk.vi"("Input Array"=u64[] []) -> ()  [unwired: 2 out]
  n228 = call <userlib>:"Search 1D Array (CXT)__ogtk.vi"("Array"=cxt[] [], "Element Data"=cxt 0.0+0.0i, "Start Index (0)"=0) -> ()  [unwired: 6 in, 1 out]
  n229 = call <userlib>:"Strip Path Extension - String__ogtk.vi"("path"="") -> ()  [unwired: 2 out]
  n230 = call <userlib>:"Reorder 2D Array2 (Boolean)__ogtk.vi"("reorder (rows)"=enum16{"rows", "columns"}."rows", "indices"=i32[] [], "array"=bool[][] []) -> ()  [unwired: 8 in, 1 out]
  n231 = call <userlib>:"Delete Elements from 2D Array (CSG)__ogtk.vi"("delete (rows or columns)"=enum16{"rows", "columns"}."rows", "indices"=i32[] [], "array"=csg[][] []) -> ()  [unwired: 7 in, 2 out]
  n232 = call <userlib>:"Remove Duplicates from 1D Array (LVObject)__ogtk.vi"("Input Array"=refnum<class>[] []) -> ()  [unwired: 2 out]
  n233 = call <userlib>:"Search 1D Array (I8)__ogtk.vi"("Array"=i8[] [], "Element Data"=i8 0, "Start Index (0)"=0) -> ()  [unwired: 6 in, 1 out]
  n234 = call <userlib>:"Strip Path Extension - 1D Array of Paths__ogtk.vi"("paths"=path[] []) -> ()  [unwired: 2 out]
  n235 = call <userlib>:"Reorder 2D Array2 (CDB)__ogtk.vi"("reorder (rows)"=enum16{"rows", "columns"}."rows", "indices"=i32[] [], "array"=cdb[][] []) -> ()  [unwired: 8 in, 1 out]
  n236 = call <userlib>:"Delete Elements from 2D Array (CXT)__ogtk.vi"("delete (rows or columns)"=enum16{"rows", "columns"}."rows", "indices"=i32[] [], "array"=cxt[][] []) -> ()  [unwired: 7 in, 2 out]
  n237 = call-poly <userlib>:"Trim Whitespace__ogtk.vi"("remove (leading and trailing)"=enum16{"leading", "trailing", "both"}."both", "String in"="") -> ()  [unwired: 5 in, 1 out]
  n238 = call <userlib>:"Search 1D Array (I16)__ogtk.vi"("Array"=i16[] [], "Element Data"=i16 0, "Start Index (0)"=0) -> ()  [unwired: 6 in, 1 out]
  n239 = call <userlib>:"Strip Path Extension - 1D Array of Strings__ogtk.vi"("paths"=string[] []) -> ()  [unwired: 2 out]
  n240 = call <userlib>:"Reorder 2D Array2 (CSG)__ogtk.vi"("reorder (rows)"=enum16{"rows", "columns"}."rows", "indices"=i32[] [], "array"=csg[][] []) -> ()  [unwired: 8 in, 1 out]
  n241 = call <userlib>:"Delete Elements from 2D Array (DBL)__ogtk.vi"("delete (rows or columns)"=enum16{"rows", "columns"}."rows", "indices"=i32[] [], "array"=dbl[][] []) -> ()  [unwired: 7 in, 2 out]
  n242 = call <userlib>:"Trim Whitespace (String)__ogtk.vi"("remove (leading and trailing)"=enum16{"leading", "trailing", "both"}."both", "String in"="") -> ()  [unwired: 5 in, 1 out]
  n243 = call <userlib>:"Search 1D Array (I32)__ogtk.vi"("Array"=i32[] [], "Element Data"=0, "Start Index (0)"=0) -> ()  [unwired: 6 in, 1 out]
  n244 = call-poly <userlib>:"Data Changed__ogtk.vi"("Variant"=variant) -> ()  [unwired: 1 out]
  n245 = call <userlib>:"Reorder 2D Array2 (CXT)__ogtk.vi"("reorder (rows)"=enum16{"rows", "columns"}."rows", "indices"=i32[] [], "array"=cxt[][] []) -> ()  [unwired: 8 in, 1 out]
  n246 = call <userlib>:"Delete Elements from 2D Array (EXT)__ogtk.vi"("delete (rows or columns)"=enum16{"rows", "columns"}."rows", "indices"=i32[] [], "array"=ext[][] []) -> ()  [unwired: 7 in, 2 out]
  n247 = call <userlib>:"Trim Whitespace (String Array)__ogtk.vi"("remove (leading and trailing)"=enum16{"leading", "trailing", "both"}."both", "String in"=string[] []) -> ()  [unwired: 5 in, 1 out]
  n248 = call <userlib>:"Search 1D Array (U8)__ogtk.vi"("Array"=u8[] [], "Element Data"=u8 0, "Start Index (0)"=0) -> ()  [unwired: 6 in, 1 out]
  n249 = call <userlib>:"Reorder 2D Array2 (DBL)__ogtk.vi"("reorder (rows)"=enum16{"rows", "columns"}."rows", "indices"=i32[] [], "array"=dbl[][] []) -> ()  [unwired: 8 in, 1 out]
  n250 = call <userlib>:"Delete Elements from 2D Array (I8)__ogtk.vi"("delete (rows or columns)"=enum16{"rows", "columns"}."rows", "indices"=i32[] [], "array"=i8[][] []) -> ()  [unwired: 7 in, 2 out]
  n251 = call <userlib>:"List Directory Recursive__ogtk.vi"("List only Top-Level files in llbs? (FALSE)"=FALSE, "error in (no error)"=errorcluster {"status"=FALSE, "code"=0, "source"=""}, "Treat llb files as directories? (FALSE)"=FALSE, "pattern"="", "Path"=path "") -> ()  [unwired: 3 in, 4 out]
  n252 = call <userlib>:"Search 1D Array (U16)__ogtk.vi"("Array"=u16[] [], "Element Data"=u16 0, "Start Index (0)"=0) -> ()  [unwired: 6 in, 1 out]
  n253 = call <userlib>:"Reorder 2D Array2 (EXT)__ogtk.vi"("reorder (rows)"=enum16{"rows", "columns"}."rows", "indices"=i32[] [], "array"=ext[][] []) -> ()  [unwired: 8 in, 1 out]
  n254 = call <userlib>:"Delete Elements from 2D Array (I16)__ogtk.vi"("delete (rows or columns)"=enum16{"rows", "columns"}."rows", "indices"=i32[] [], "array"=i16[][] []) -> ()  [unwired: 7 in, 2 out]
  n255 = call-poly <userlib>:"Filter 1D Array__ogtk.vi"("items to filter"=dbl[] [], "array"=dbl[] []) -> ()  [unwired: 4 in, 2 out]
  n256 = call <userlib>:"Search 1D Array (U32)__ogtk.vi"("Array"=u32[] [], "Element Data"=u32 0, "Start Index (0)"=0) -> ()  [unwired: 6 in, 1 out]
  n257 = call <userlib>:"Reorder 2D Array2 (I8)__ogtk.vi"("reorder (rows)"=enum16{"rows", "columns"}."rows", "indices"=i32[] [], "array"=i8[][] []) -> ()  [unwired: 8 in, 1 out]
  n258 = call <userlib>:"Search 1D Array (Boolean)__ogtk.vi"("Array"=bool[] [], "Element Data"=FALSE, "Start Index (0)"=0) -> ()  [unwired: 6 in, 1 out]
  n259 = call <userlib>:"Reorder 2D Array2 (I16)__ogtk.vi"("reorder (rows)"=enum16{"rows", "columns"}."rows", "indices"=i32[] [], "array"=i16[][] []) -> ()  [unwired: 8 in, 1 out]
  n260 = call <userlib>:"Reorder 2D Array2 (I32)__ogtk.vi"("reorder (rows)"=enum16{"rows", "columns"}."rows", "indices"=i32[] [], "array"=i32[][] []) -> ()  [unwired: 8 in, 1 out]
  n261 = call <userlib>:"Reorder 2D Array2 (Path)__ogtk.vi"("reorder (rows)"=enum16{"rows", "columns"}."rows", "indices"=i32[] [], "array"=path[][] []) -> ()  [unwired: 8 in, 1 out]
  n262 = call <userlib>:"Reorder 2D Array2 (SGL)__ogtk.vi"("reorder (rows)"=enum16{"rows", "columns"}."rows", "indices"=i32[] [], "array"=sgl[][] []) -> ()  [unwired: 8 in, 1 out]
  n263 = call <userlib>:"Reorder 2D Array2 (String)__ogtk.vi"("reorder (rows)"=enum16{"rows", "columns"}."rows", "indices"=i32[] [], "array"=string[][] []) -> ()  [unwired: 8 in, 1 out]
  n264 = call <userlib>:"Reorder 2D Array2 (U8)__ogtk.vi"("reorder (rows)"=enum16{"rows", "columns"}."rows", "indices"=i32[] [], "array"=u8[][] []) -> ()  [unwired: 8 in, 1 out]
  n265 = call <userlib>:"Reorder 2D Array2 (U16)__ogtk.vi"("reorder (rows)"=enum16{"rows", "columns"}."rows", "indices"=i32[] [], "array"=u16[][] []) -> ()  [unwired: 8 in, 1 out]
  n266 = call <userlib>:"Reorder 2D Array2 (U32)__ogtk.vi"("reorder (rows)"=enum16{"rows", "columns"}."rows", "indices"=i32[] [], "array"=u32[][] []) -> ()  [unwired: 8 in, 1 out]
